vi "Connect Meas Plugin APIs.vi"(0 "Logic VI Ref":refnum<vi>, 5 "SubVIs":refnum<vi>[](array[refnum]), 11 "error in (no error)":errorcluster) -> (15 "error out":errorcluster)   [LabVIEW 2021, in "Migrator.lvlib"]
uses:
  Migrator.lvlib
  Migrator Reusables/Migrator Reusables.lvlib
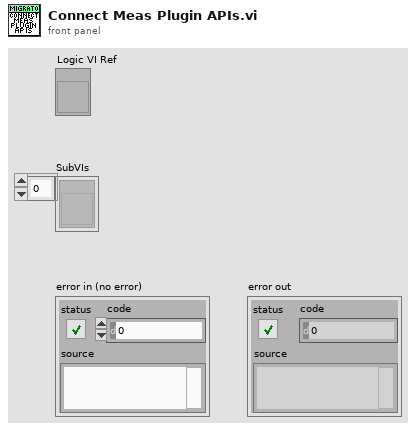
[diagram p1: front panel]
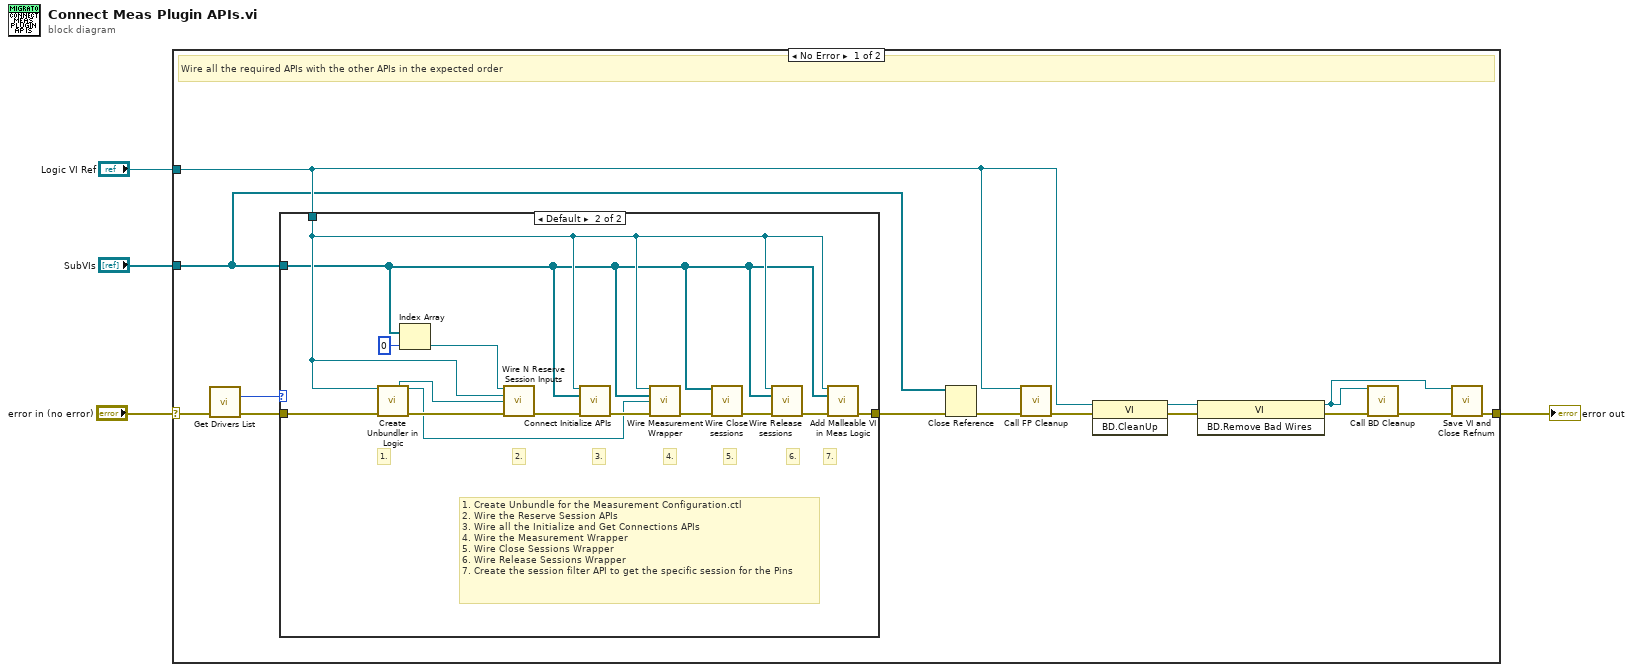
[diagram p0: block diagram]
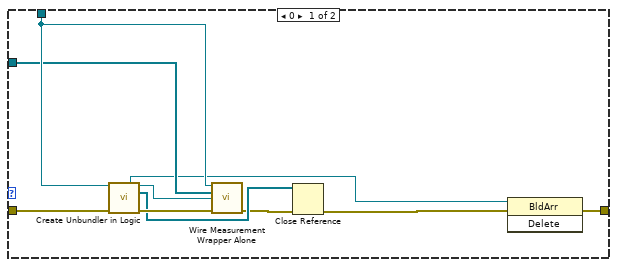
[diagram p2: hidden frame]
diagram:
  n1 = case shown="No Error" "error in (no error)" {
    selector: "error in (no error)" -> [w17 w42]
    tunnel: "Logic VI Ref" -> [w13 _]
    tunnel: "SubVIs" -> [w11 _]
    tunnel: [w16 w42] -> w1
    frame No Error {
      # "Wire all the required APIs with the other APIs in the expected order"
      n2 = call "Get Drivers List.vi"() -> ("Total Driver List"=w9:i32)  [unwired: 10 in, 5 out]
      n3 = case shown="Default" w9 {
        tunnel: w17 -> [w26 w41]
        tunnel: w13 -> [w24 w29]
        tunnel: [w21 w30] -> w12
        tunnel: w11 -> [w23 w28]
        frame 0 {
          n4 = call "Create Unbundler in Logic.vi"("VI in"=w24, "error in (no error)"=w26) -> ("Build Array Ref"=w22:refnum<vi>, "Configration Terminal"=w27:refnum<vi>, "Unbundle OutputTerms[]"=w20:refnum<vi>[], "error out"=w25:errorcluster)  [unwired: 10 in]
          n5 = call "Wire Measurement Wrapper Alone.vi"("vi reference"=w24, "SubVI in"=w23, "Terminal"=w27, "error in (no error)"=w25) -> ("error out"=w18:errorcluster)  [unwired: 11 in]
          n6 = Close Reference(reference=w20, error in (no error)=w18) -> (error out=w19:errorcluster)
          n7 = invoke class="BldArr" method="Delete"(reference=w22, error in=w19) -> (error out=w21:errorcluster)  [unwired: 1 in, 2 out]
        }
        frame Default {
          # "1. Create Unbundle for the Measurement Configuration.ctl\n2. Wire the Reserve Session APIs\n3. Wire all the Initialize and Get Connections APIs\n4. Wire the Measurement Wrapper\n5. Wire Close Sessions Wrapper\n6. Wire Release Sessions Wrapper\n7. Create the session filter API to get the specific session for the Pins"
          # "7."
          # "6."
          # "5."
          # "4."
          # "3."
          # "2."
          # "1."
          n8 = call "Create Unbundler in Logic.vi"("VI in"=w29, "error in (no error)"=w41) -> ("Build Array Ref"=w37:refnum<vi>, "Configration Terminal"=w33:refnum<vi>, "error out"=w38:errorcluster)  [unwired: 10 in, 1 out]
          n9 = Index Array(array=w28, index=0) -> (element=w39:refnum<vi>)
          n10 = call "Wire N Reserve Session Inputs.vi"("SubVI in"=w39, "vi reference"=w29, "Build Array"=w37, "error in (no error)"=w38) -> ("error out"=w32:errorcluster)  [unwired: 11 in]
          n11 = call "Connect Initialize APIs.vi"("Logic VI Ref"=w29, "SubVIs"=w28, "error in (no error)"=w32) -> ("error out"=w36:errorcluster)  [unwired: 12 in]
          n12 = call "Wire Measurement Wrapper.vi"("vi reference"=w29, "SubVI in"=w28, "Terminal"=w33, "error in (no error)"=w36) -> ("error out"=w35:errorcluster)  [unwired: 11 in]
          n13 = call "Wire Close sessions.vi"("SubVIs Ref"=w28, "error in (no error)"=w35) -> ("error out"=w34:errorcluster)  [unwired: 13 in]
          n14 = call "Wire Release sessions.vi"("Logiv VI Ref"=w29, "SubVIs Ref"=w28, "error in"=w34) -> ("error out"=w31:errorcluster)  [unwired: 12 in]
          n15 = call "Add Malleable VI in Meas Logic.vi"("Logic VI"=w29, "SubVIs Ref"=w28, "error in (no error)"=w31) -> ("error out"=w30:errorcluster)  [unwired: 12 in]
        }
      }
      n16 = Close Reference(reference=w11, error in (no error)=w12) -> (error out=w15:errorcluster)
      n17 = call "Call FP Cleanup.vi"("VI"=w13, "error in (no error)"=w15) -> ("error out"=w14:errorcluster)  [unwired: 13 in]
      n18 = invoke class="VI" method="BD.CleanUp"(reference=w13, error in=w14) -> (reference out=w8:refnum<vi>, error out=w5:errorcluster)  [unwired: 1 in, 1 out]
      n19 = invoke class="VI" method="BD.Remove Bad Wires"(reference=w8, error in=w5) -> (reference out=w7:refnum<vi>, error out=w6:errorcluster)  [unwired: 1 in, 1 out]
      n20 = call "Call BD Cleanup.vi"("VI"=w7, "error in (no error)"=w6) -> ("error out"=w10:errorcluster)  [unwired: 13 in]
      n21 = call "Save VI and Close Refnum.vi"("VI Refnum"=w7, "error in"=w10) -> ("error out"=w16:errorcluster)  [unwired: 13 in]
    }
    frame Error {
    }
  }
  "error out" <- w1
